vi "Caller.vi"(6 "Sub Panel":refnum<vi>, 8 "Error In":errorcluster, 10 "Data Value Reference In":refnum<data-value>, 11 "Multiply In":refnum<class "Multiply.lvclass">) -> (0 "Error Out":errorcluster, 3 "Multiply Out":refnum<class "Multiply.lvclass">)   [LabVIEW 2021, in "Calculator.lvlib" / "Multiply.lvclass"]
doc: "This VI is an overriding method , which asynchronously calls the UI.vi ."
uses:
  Multiply.lvclass
  UI.vi
  NumericOperation/NumericOperation.lvclass
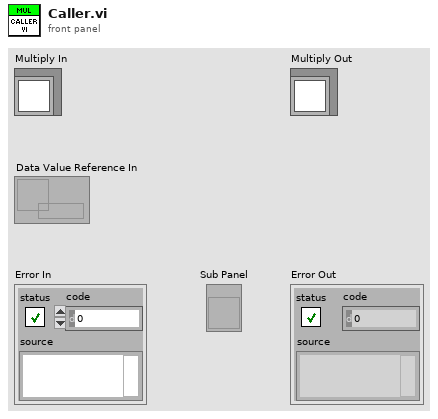
[diagram p1: front panel]
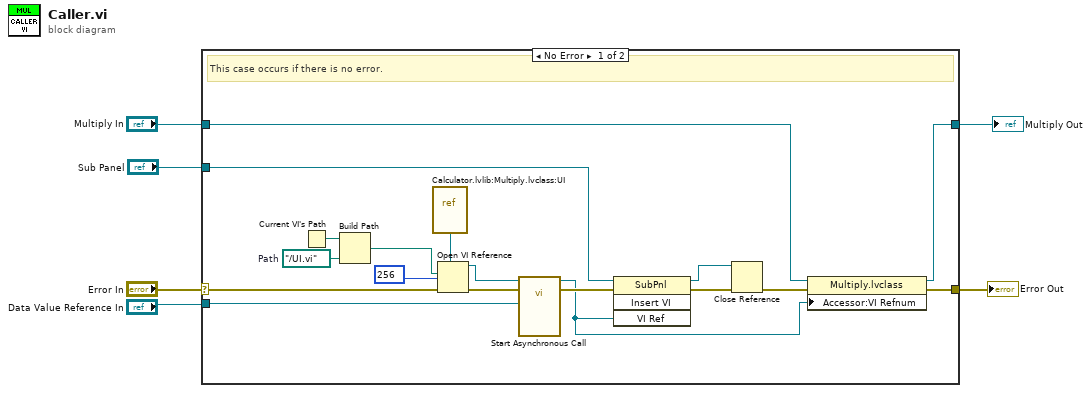
[diagram p0: block diagram]
diagram:
  n1 = case shown="No Error" "Error In" {
    selector: "Error In" -> [w24 w26]
    tunnel: [w13 w26] -> w5
    tunnel: [w10 w25] -> w3
    tunnel: "Multiply In" -> [w12 w25]
    tunnel: "Sub Panel" -> [w15 _]
    tunnel: "Data Value Reference In" -> [w7 _]
    frame No Error {
      w20 = path "../UI.vi"  # Path
      # "This case occurs if there is no error."
      n2 = Current VI's Path() -> (path=w21:path)
      n3 = Build Path(base path=w21, name or relative path=w20) -> (appended path=w19:path)
      n4 = vi-ref "Calculator.lvlib:Multiply.lvclass:UI.vi"() -> (w18:refnum<vi>)
      n5 = Open VI Reference(type specifier VI Refnum (for type only)=w18, vi path=w19, options=256, error in (no error)=w24) -> (vi reference=w17:refnum<vi>, error out=w23:errorcluster)  [unwired: 2 in]
      n6 = call-by-ref "Start Asynchronous Call"(reference=w17, error in=w23, "Data Value Reference In"=w7) -> (reference out=w11:refnum<vi>, error out=w22:errorcluster)  [unwired: 8 in, 3 out]
      n7 = invoke class="SubPnl" method="Insert VI"(reference=w15, error in=w22, "VI Ref"=w11) -> (reference out=w8:refnum<vi>, error out=w16:errorcluster)  [unwired: 1 in, 2 out]
      n8 = Close Reference(reference=w8, error in (no error)=w16) -> (error out=w9:errorcluster)
      n9 = property class="Multiply.lvclass"(reference=w12, error in=w9, "Accessor:VI Refnum"=w11) -> (reference out=w10:refnum<class "Multiply.lvclass">, error out=w13:errorcluster)
    }
    frame Error {
      # "This case occurs if there is any error."
    }
  }
  "Error Out" <- w5
  "Multiply Out" <- w3
